vi "Global_Bin_Out_Mode.vi"() -> ()   [LabVIEW 2016, in "DNP3_Master_Station_Template.lvlib"]
uses:
  <vilib>/DNP3/DNP3_Master/Operation Mode.ctl
  DNP3_Master_Station_Template.lvlib
  <vilib>/DNP3/DNP3_Master.lvlib
panel:
  in  "Binary Out Mode":T1=6 items=["SBO"=0, "Select"=3, "Operate"=4, "Direct"=5, "Direct No Ack"=6]
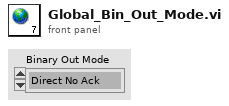
[diagram p1: front panel]
types:
  T1 = typedef "DNP3_Master.lvlib/Operation Mode.ctl" = u8
diagram:
